vi "ge_DAQMain.vi"(8 "error in":errorcluster, 11 "DaqQ Name":string) -> (0 "error IO":errorcluster)   [LabVIEW 2012]
uses:
  Custom Ctrls/ge_TaskModBus.ctl
  Custom Ctrls/ge_AMC_Qname.ctl
  <resource>/objmgr/daqmx.rc
  Classes/Data Acquisition/Class DAQ Actor/DAQ Actor.lvclass
  Common/Controls/Group Timing Info.ctl
  Common/Controls/TE_Designator.ctl
  SubVIs Main/SubVIs DAQ/Custom Ctrls/ge_DAQBlockInfo.ctl
  SubVIs Main/SubVIs DAQ/Custom Ctrls/ge_DAQGrandmaster.ctl
  SubVIs Main/EZ Msg/ezm_Message.ctl
  <vilib>/DAQmx/read.llb/DAQmx Read (Analog 1D Wfm NChan NSamp).vi
  SubVIs Main/SubVIs DAQ/Custom Ctrls/ge_ThreadDiag.ctl
  <vilib>/addons/internet/NI_InternetTK_Core_VIs.lvlib
  Classes/Measurements/Class Channel/Channel.lvclass
panel:
  out "Numeric":i32
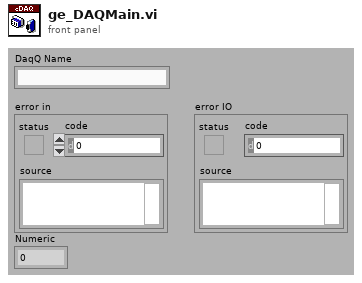
[diagram p1: front panel]
types:
  T1 = typedef "ge_DAQGrandmaster.ctl" = cluster{"Blocks ID":u32, "SisterThreadQName":string, "Chassis Name":string, "IP Address":string, "Speed":T2, "Backlog ID":string, "Backlog Enable":bool, "AllChans":refnum<class "Channel.lvclass">[], "ScalPrevNot":refnum<notifier>, "WfmPrevNot":refnum<notifier>, "DAQmx Task":refnum<k21>, "DS Conn":refnum<k13>, "DAQBlockInfo":T3, "TCP Wfm Queue":refnum<queue>, "UI Queue":refnum<queue>, "LS TCP Wfm Queue":refnum<queue>}
  T2 = typedef "TE_Designator.ctl" = enum16{"High Speed", "Low Speed"}
  T3 = typedef "ge_DAQBlockInfo.ctl" = cluster{"SampRate":dbl, "BufSize":u32, "ReadBlk":i32, "TCP Gap":i32}
  T4 = typedef "ge_AMC_Qname.ctl" = enum16{"Cmnd Loop", "UI Updater", "Conn Mgr HS", "Conn Mgr LS", "TCP Send HS", "TCP Send LS"}
  T5 = enum16{"Read", "Write", "ReadWrite", "BufferedRead", "BufferedReadWrite"}
  T6 = typedef "ge_ThreadDiag.ctl" = cluster{"Loop It":i32, "LoopRate (ms)":u32, "Bff Bcklg":dbl}
  T7 = typedef "ge_TaskModBus.ctl" = cluster{"Modbus URL":string, "Task":refnum<k21>, "IP Address":string, "GrpCfg":T8}
  T8 = typedef "Group Timing Info.ctl" = cluster{"Rate":dbl, "ReadBlk":i32, "TCP Gap":i32}
  T9 = typedef "DAQ Task Role.ctl" = enum16{"Master", "Slave", "Stand Alone", "None"}
  T10 = typedef "Telnet Session.ctl" = refnum<k1>
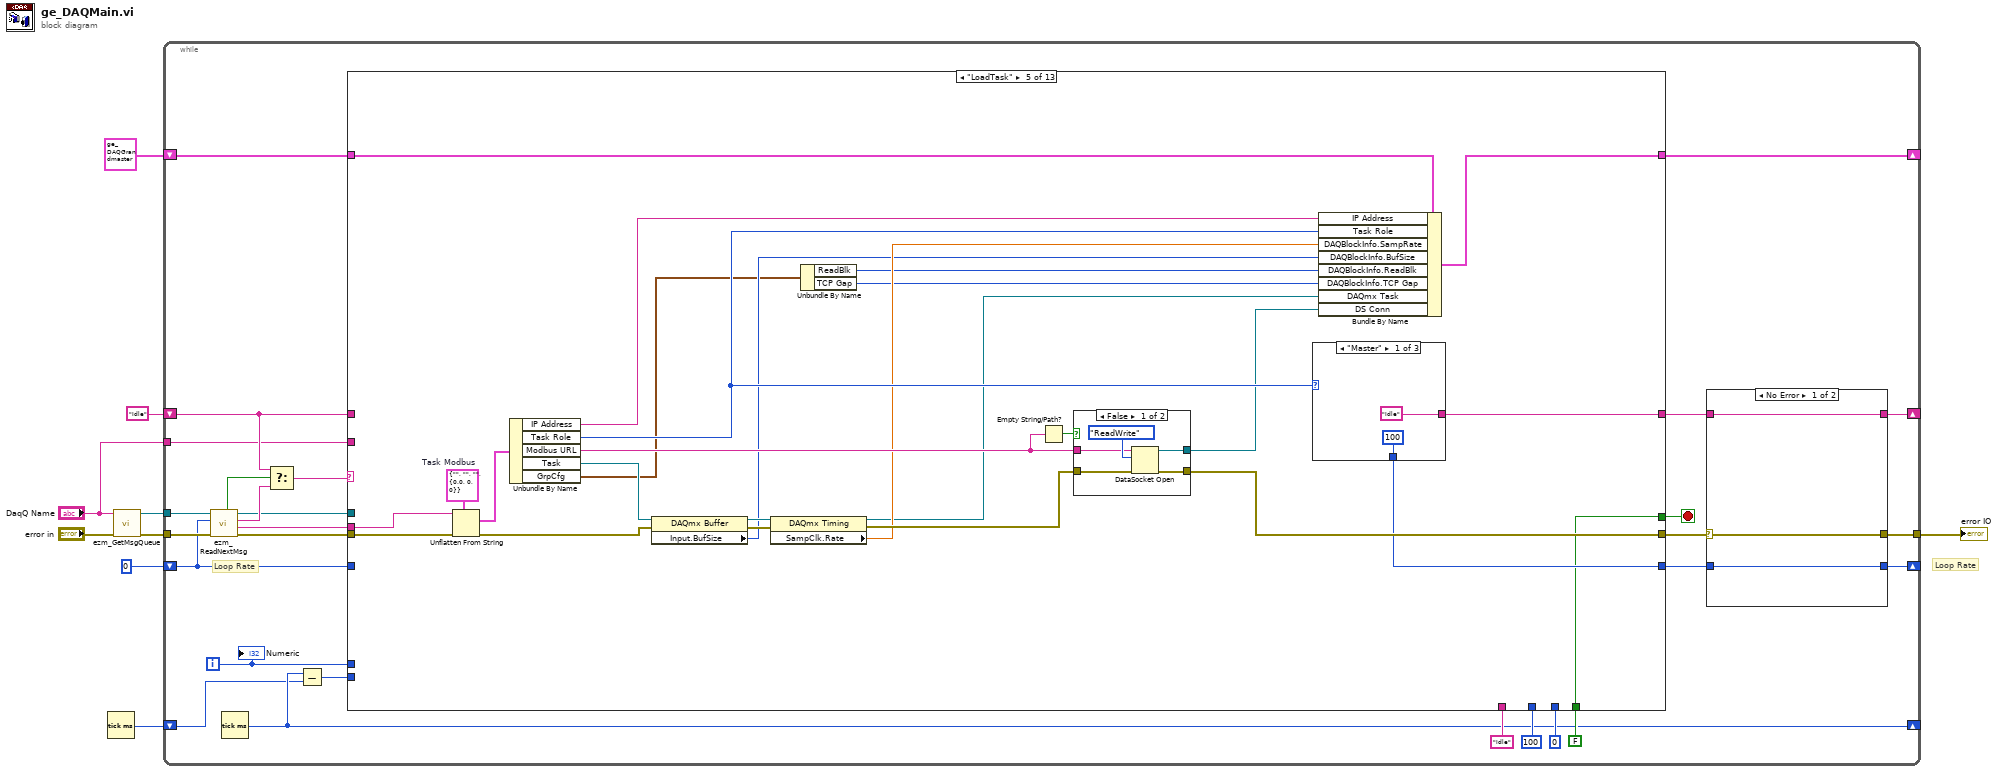
[diagram p0: block diagram]
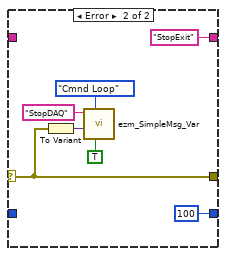
[diagram p2: hidden frame]
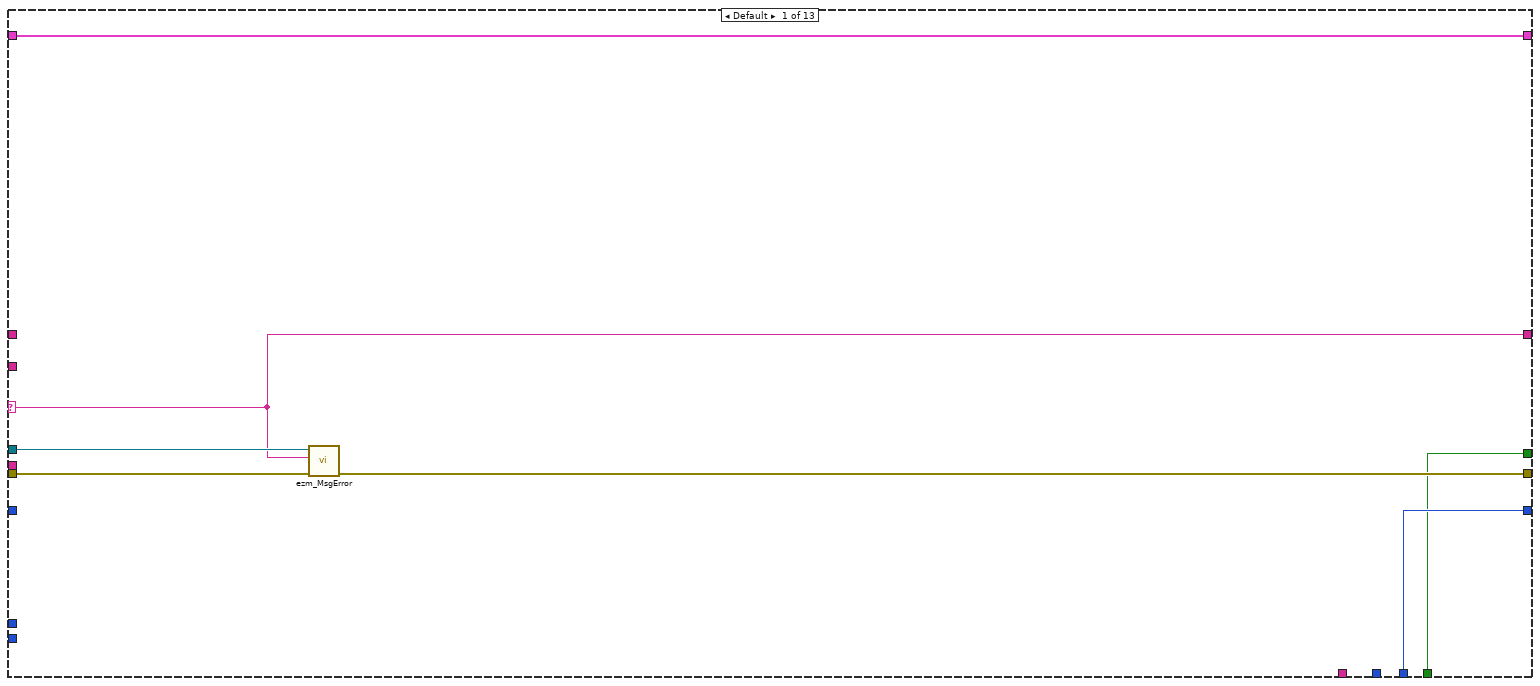
[diagram p3: hidden frame]
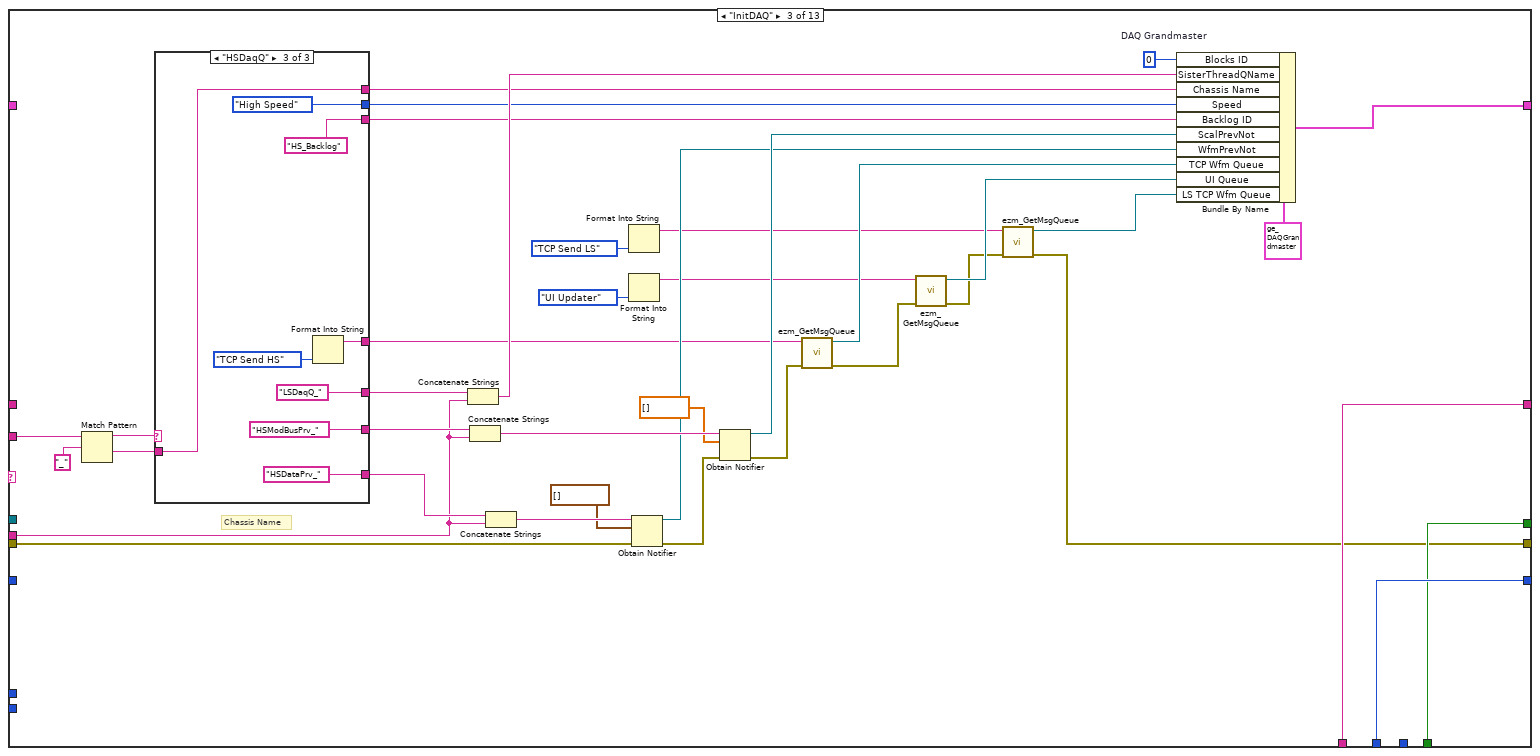
[diagram p5: hidden frame]
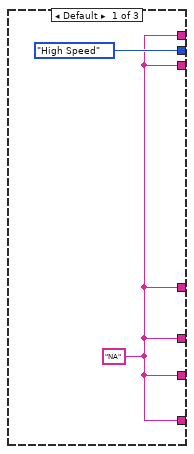
[diagram p6: hidden frame]
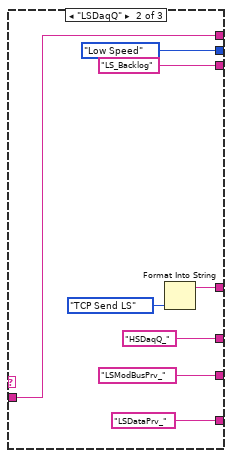
[diagram p7: hidden frame]
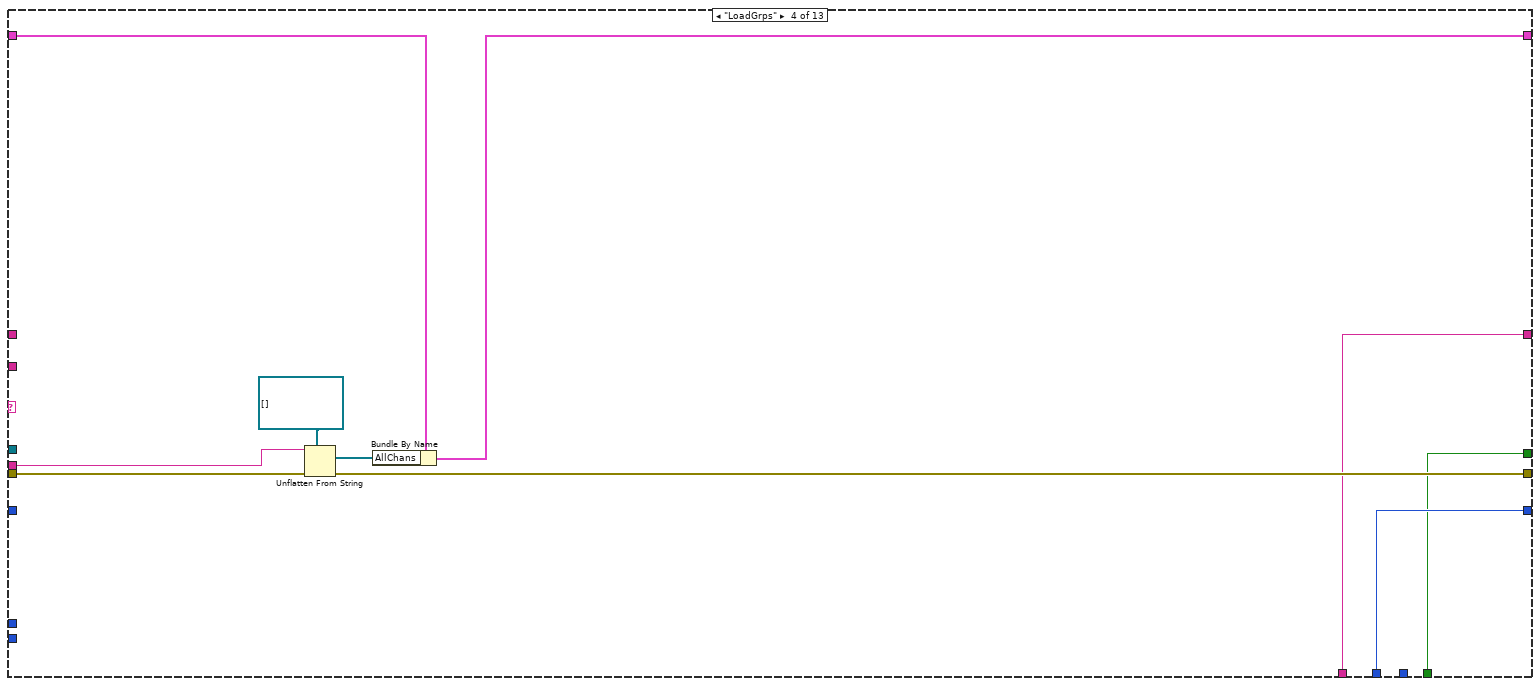
[diagram p8: hidden frame]
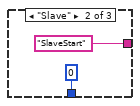
[diagram p9: hidden frame]
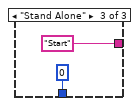
[diagram p10: hidden frame]
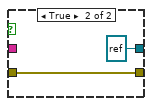
[diagram p11: hidden frame]
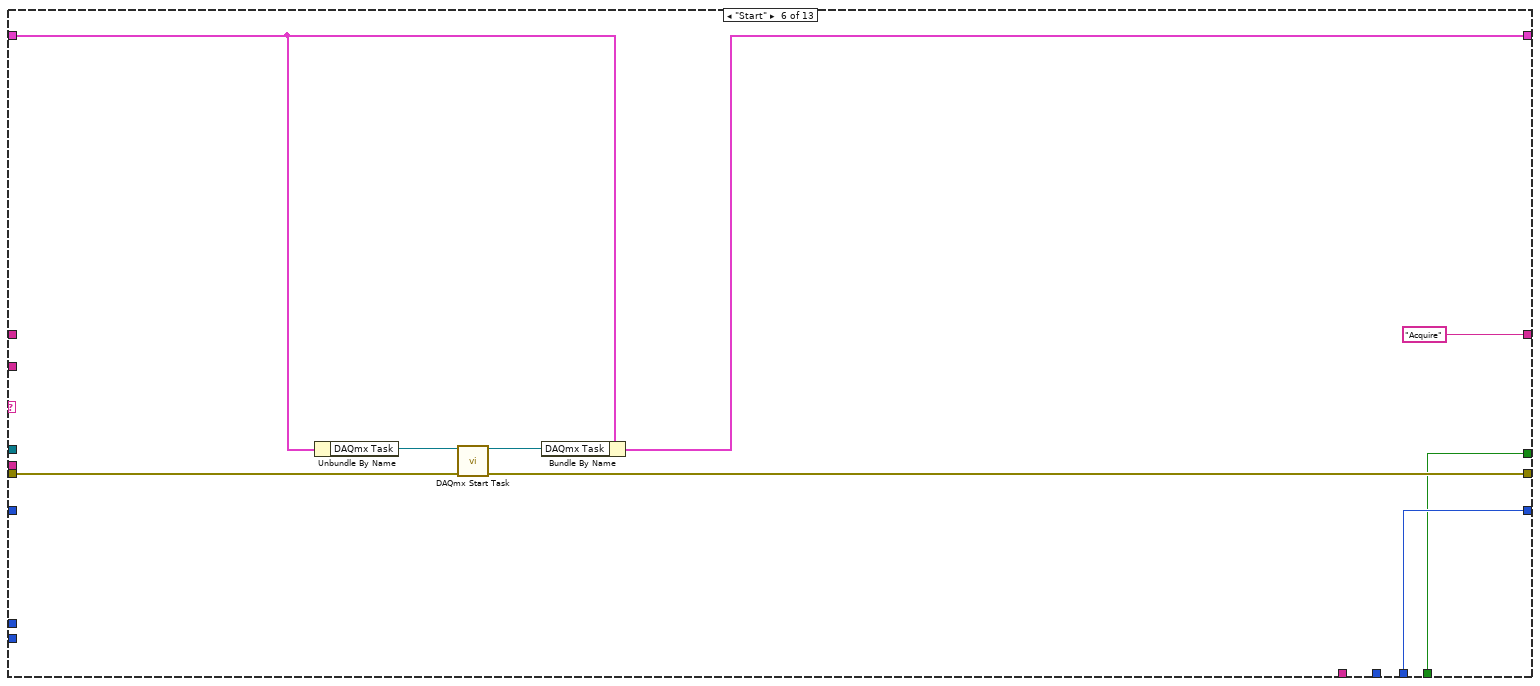
[diagram p12: hidden frame]
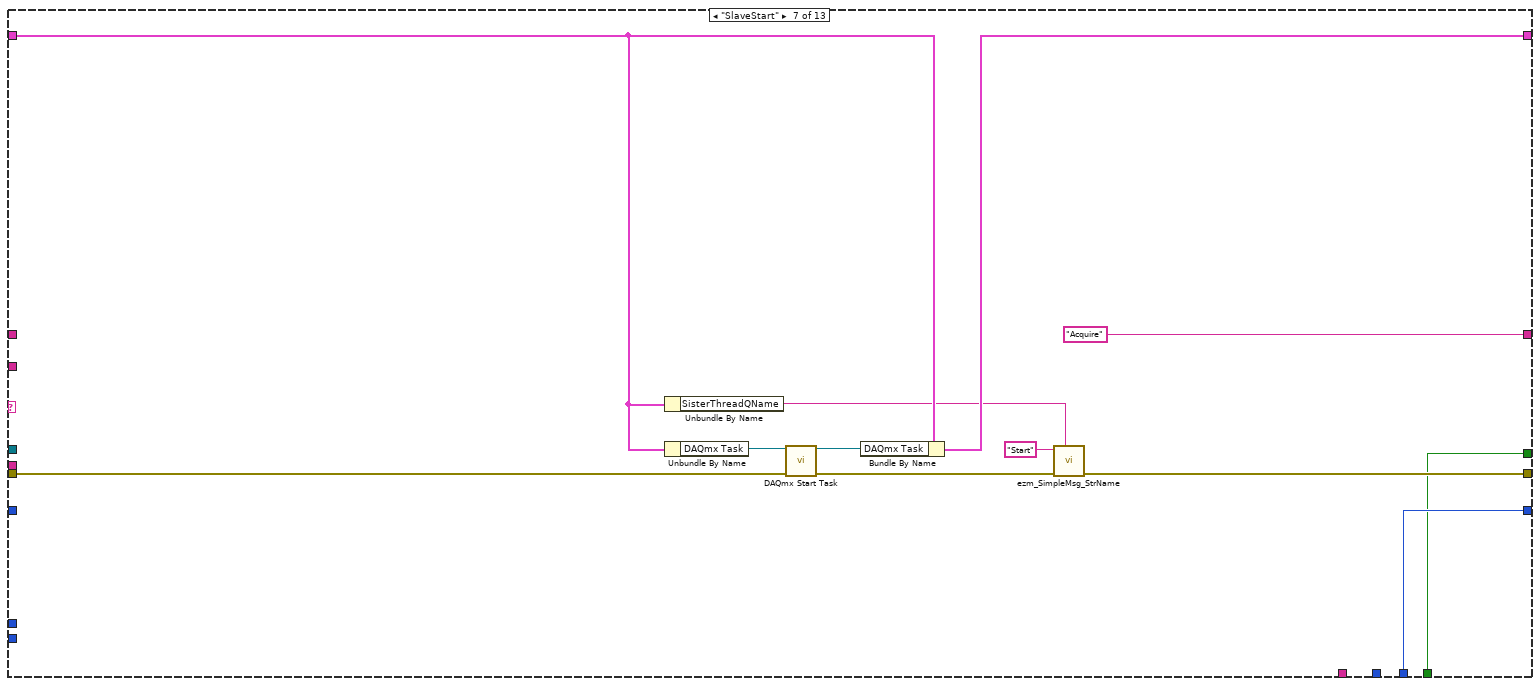
[diagram p13: hidden frame]
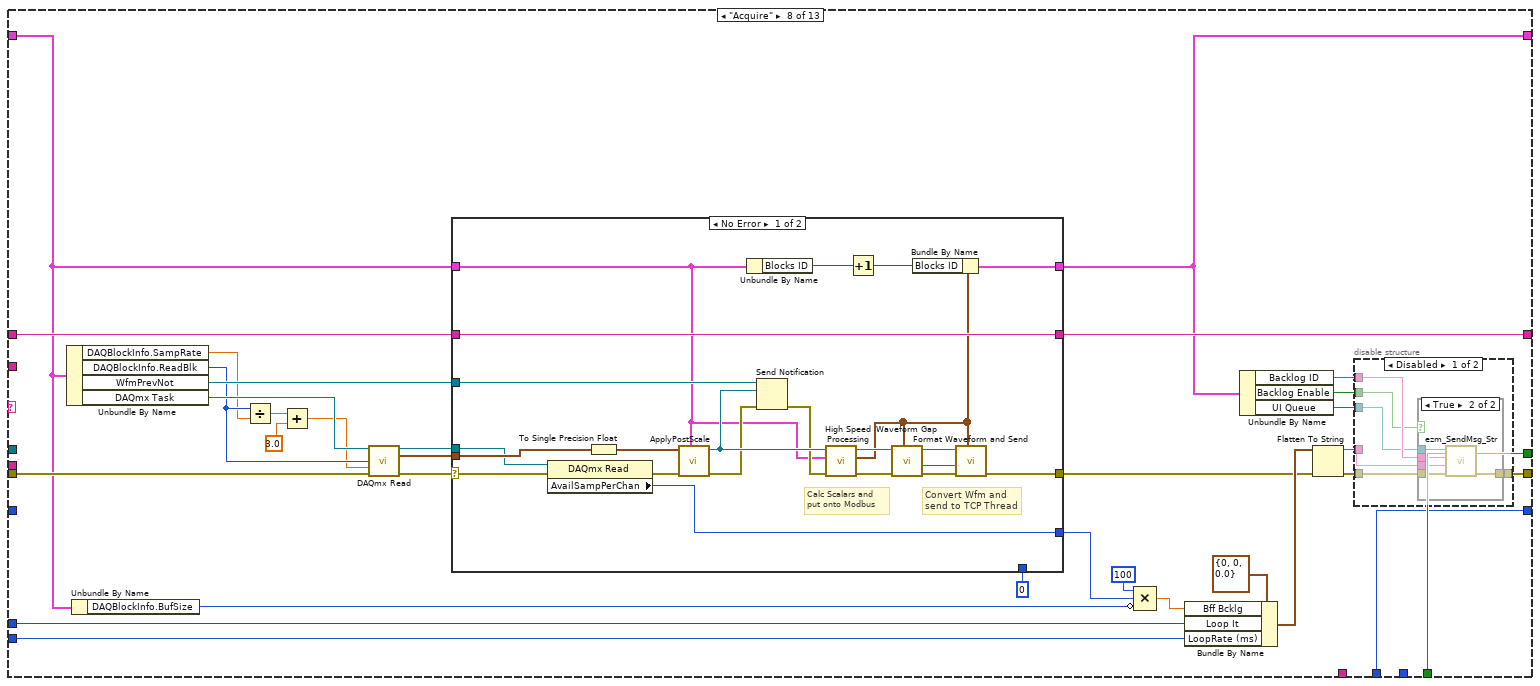
[diagram p14: hidden frame]
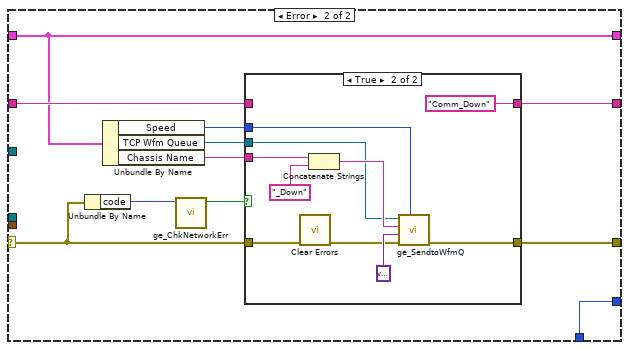
[diagram p17: hidden frame]
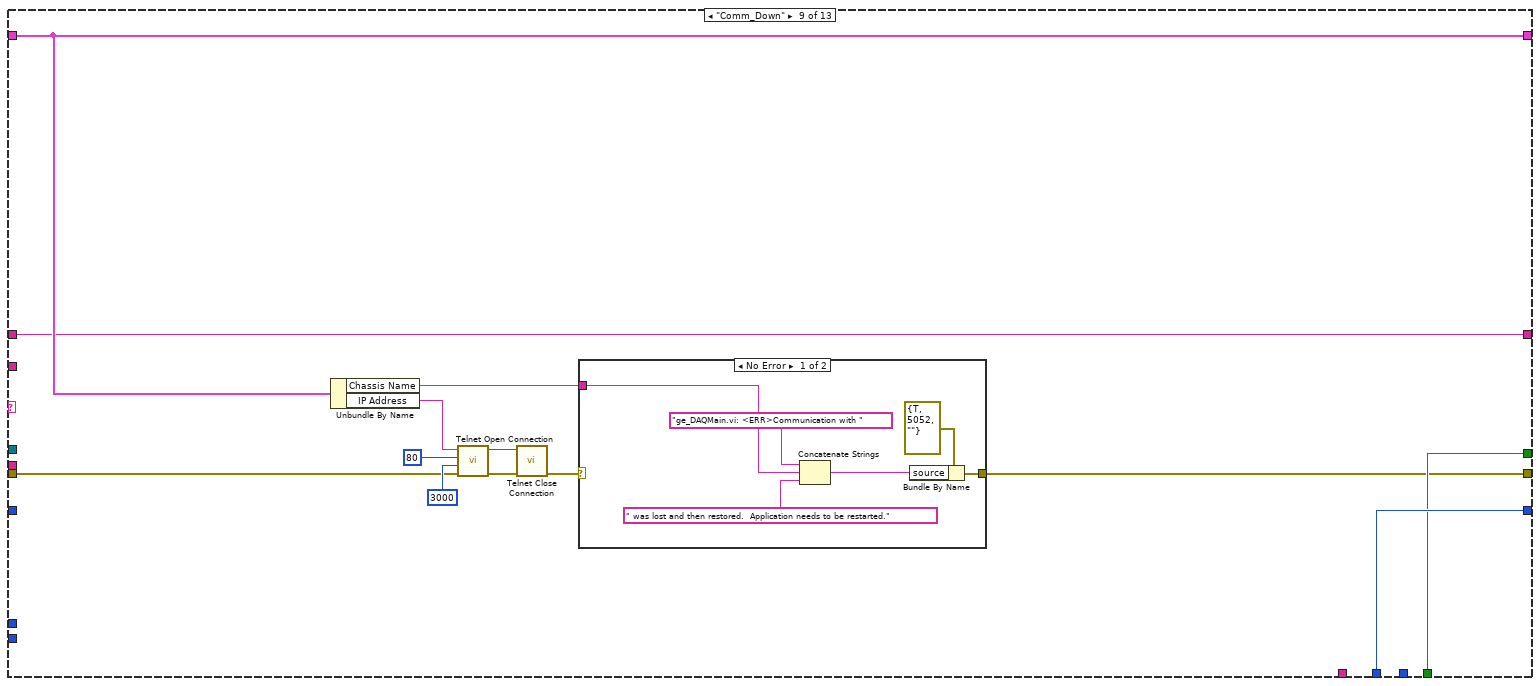
[diagram p19: hidden frame]
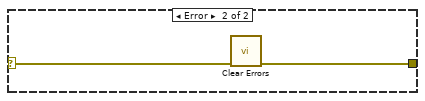
[diagram p20: hidden frame]
diagram:
  # "Loop Rate"
  n1 = Tick Count (ms)() -> (millisecond timer value=w3:u32)
  n2 = call "ezm_GetMsgQueue.vi"("error in"="error in", "Queue Name"="DaqQ Name") -> ("error out"=w6:errorcluster, "queue out"=w5:refnum<queue>)  [unwired: 8 in]
  n3 = while {
    tunnel: w6 -> [w36]
    tunnel: w5 -> [w37]
    shift-right: [w25] -> _
    shift-left: "Idle" ("Message Queue Name") -> [w21]
    shift-right: [w26] -> _
    shift-left: u32 0 -> [w30]
    tunnel: [w23] -> w2
    tunnel: "DaqQ Name" -> [w20]
    shift-right: [w15] -> _
    shift-left: T1 {"Blocks ID"=0, "SisterThreadQName"="", "Chassis Name"="", "IP Address"="", "Speed"=enum."High Speed", "Backlog ID"="", "Backlog Enable"=FALSE, "AllChans"=[], "ScalPrevNot"=refnum, "WfmPrevNot"=refnum, "DAQmx Task"="", "DS Conn"=refnum, "DAQBlockInfo"={"SampRate"=0.0, "BufSize"=0, "ReadBlk"=0, "TCP Gap"=0}, "TCP Wfm Queue"=refnum, "UI Queue"=refnum, "LS TCP Wfm Queue"=refnum} ("DAQ Grandmaster Out") -> [w14]
    shift-right: [w13] -> _
    shift-left: w3 -> [w12]
    i -> [w10]
    stop <- w17 stop-if-true
    # "Loop Rate"
    n4 = call "ezm_ReadNextMsg.vi"("error in"=w36, "timeout (0ms)"=w30, "Msg Queue In"=w37) -> ("error out"=w32:errorcluster, "Msg Value"=w33:string, "Msg Name"=w31:string, "Msg Queue Out"=w29:refnum<queue>, "timed out?"=w18:bool)  [unwired: 2 in, 2 out]
    n5 = Tick Count (ms)() -> (millisecond timer value=w13:u32)
    n6 = Select(t=w21, s=w18, f=w31) -> (s? t:f=w19:string)
    n7 = Subtract(x=w13, y=w12) -> (x-y=w11:u32)
    n8 = case shown="\"LoadTask\"" w19 {
      selector: w19 -> [w50 _ _ _ _ _ _ _ _ _ _ _ _]
      tunnel: w32 -> [w54 w59 w94 w124 w150 w173 w185 w209 w282 w303 w310 w329 w363]
      tunnel: [w53 w59 w63 w123 w141 w172 w182 w218 w287 w303 w310 w328 w383] -> w28
      tunnel: [w52 w58 w97 w121 w138 w170 w183 w203 w289 w302 w309 w324 u32 1000] -> w27
      tunnel: u32 0 -> [w52 _ _ _ _ w170 w183 _ _ _ _ w323 _]
      tunnel: w33 -> [_ _ w82 w125 w151 _ _ _ _ _ _ _ _]
      tunnel: u32 100 -> [_ w58 w97 w121 _ _ _ w203 w289 _ _ _ _]
      tunnel: [w50 w57 w90 w122 w148 "Acquire" ("Msg Name") "Acquire" ("Msg Name") w199 w285 w304 w311 w325 w382] -> w24
      tunnel: w30 -> [_ _ _ _ _ _ _ _ _ w302 w309 _ _]
      tunnel: w29 -> [w51 _ _ _ _ _ _ _ _ _ _ w330 w384]
      tunnel: "Idle" ("Msg Name") -> [_ w57 w90 w122 _ _ _ _ _ _ _ w326 w382]
      tunnel: w21 -> [_ _ _ _ _ _ _ w198 w285 w304 w311 w327 _]
      tunnel: w20 -> [_ _ w86 _ _ _ _ _ _ _ _ _ _]
      tunnel: [w49 w56 w81 w120 w137 w169 w179 w217 w288 w301 w308 w321 TRUE] -> w17
      tunnel: FALSE -> [w49 w56 w81 w120 w137 w169 w179 w217 w288 w301 w308 w322 _]
      tunnel: [w48 w55 w78 w118 w135 w165 w176 w190 w286 w298 w305 w320 w376] -> w15
      tunnel: w14 -> [w48 w55 _ w119 w136 w167 w175 w191 w286 w299 w306 w320 w376]
      tunnel: w11 -> [_ _ _ _ _ _ _ w212 _ _ _ _ _]
      tunnel: w10 -> [_ _ _ _ _ _ _ w210 _ _ _ _ _]
      frame Default {
        n9 = call "ezm_MsgError.vi"("error in"=w54, "AMC Msg Name"=w50, "Msg Queue"=w51) -> ("error out"=w53:errorcluster)  [unwired: 8 in]
      }
      frame "Idle" {
      }
      frame "InitDAQ" {
        w80 = T1 {"Blocks ID"=0, "SisterThreadQName"="", "Chassis Name"="", "IP Address"="", "Speed"=enum."High Speed", "Backlog ID"="", "Backlog Enable"=FALSE, "AllChans"=[], "ScalPrevNot"=refnum, "WfmPrevNot"=refnum, "DAQmx Task"="", "DS Conn"=refnum, "DAQBlockInfo"={"SampRate"=0.0, "BufSize"=0, "ReadBlk"=0, "TCP Gap"=0}, "TCP Wfm Queue"=refnum, "UI Queue"=refnum, "LS TCP Wfm Queue"=refnum}  # DAQ Grandmaster
        # "Chassis Name"
        n10 = Match Pattern(string=w86, regular expression="_") -> (before substring=w85:string, after substring=w84:string)  [unwired: 1 in, 2 out]
        n11 = case shown="\"HSDaqQ\"" w85 {
          tunnel: [w98 "LS_Backlog" ("Msg Name") "HS_Backlog" ("Msg Name")] -> w72
          tunnel: [w98 "LSModBusPrv_" ("name (unnamed)") "HSModBusPrv_" ("name (unnamed)")] -> w89
          tunnel: [w98 "LSDataPrv_" ("name (unnamed)") "HSDataPrv_" ("name (unnamed)")] -> w88
          tunnel: w84 -> [_ w103 w111]
          tunnel: [w98 w103 w111] -> w73
          tunnel: [TE_Designator."High Speed" ("Rate") TE_Designator."Low Speed" ("Rate") TE_Designator."High Speed" ("Rate")] -> w76
          tunnel: [w98 "HSDaqQ_" "LSDaqQ_"] -> w83
          tunnel: [w98 w100 w108] -> w69
          frame Default {
            w98 = "NA" ("Msg Name")
          }
          frame "LSDaqQ" {
            n12 = Format Into String(ge_AMC_Qname."TCP Send LS" ("ge_AMC_Qname")) -> (resulting string=w100:string)  [unwired: 3 in, 1 out]
          }
          frame "HSDaqQ" {
            n13 = Format Into String(ge_AMC_Qname."TCP Send HS" ("ge_AMC_Qname")) -> (resulting string=w108:string)  [unwired: 3 in, 1 out]
          }
        }
        n14 = Concatenate Strings(w83, w82) -> (w77:string)
        n15 = Concatenate Strings(w89, w82) -> (w92:string)
        n16 = Concatenate Strings(w88, w82) -> (w96:string)
        n17 = Format Into String(ge_AMC_Qname."TCP Send LS" ("ge_AMC_Qname")) -> (resulting string=w61:string)  [unwired: 3 in, 1 out]
        n18 = Format Into String(ge_AMC_Qname."UI Updater" ("ge_AMC_Qname")) -> (resulting string=w67:string)  [unwired: 3 in, 1 out]
        n19 = Obtain Notifier(name (unnamed)=w96, notification data type=waveform(sgl)[] [] ("data"), error in (no error)=w94) -> (notifier out=w74:refnum<notifier>, error out=w93:errorcluster)  [unwired: 1 in, 1 out]
        n20 = Obtain Notifier(name (unnamed)=w92, notification data type=dbl[] [], error in (no error)=w93) -> (notifier out=w75:refnum<notifier>, error out=w71:errorcluster)  [unwired: 1 in, 1 out]
        n21 = call "ezm_GetMsgQueue.vi"("error in"=w71, "Queue Name"=w69) -> ("error out"=w66:errorcluster, "queue out"=w70:refnum<queue>)  [unwired: 8 in]
        n22 = call "ezm_GetMsgQueue.vi"("error in"=w66, "Queue Name"=w67) -> ("error out"=w64:errorcluster, "queue out"=w65:refnum<queue>)  [unwired: 8 in]
        n23 = call "ezm_GetMsgQueue.vi"("error in"=w64, "Queue Name"=w61) -> ("error out"=w63:errorcluster, "queue out"=w60:refnum<queue>)  [unwired: 8 in]
        n24 = Bundle By Name(cluster=w80, "Blocks ID"=u32 0, "SisterThreadQName"=w77, "Chassis Name"=w73, "Speed"=w76, "Backlog ID"=w72, "ScalPrevNot"=w75, "WfmPrevNot"=w74, "TCP Wfm Queue"=w70, "UI Queue"=w65, "LS TCP Wfm Queue"=w60) -> (w78:T1)
      }
      frame "LoadGrps" {
        n25 = Unflatten From String(type=refnum<class "Channel.lvclass">[] [] ("AllChans"), binary string=w125, error in (no error)=w124) -> (value=w116:refnum<class "Channel.lvclass">[], error out=w123:errorcluster)  [unwired: 2 in, 1 out]
        n26 = Bundle By Name(cluster=w119, "AllChans"=w116) -> (w118:T1)
      }
      frame "LoadTask" {
        w149 = T7 {"Modbus URL"="", "Task"="", "IP Address"="", "GrpCfg"={"Rate"=0.0, "ReadBlk"=0, "TCP Gap"=0}}  # Task Modbus
        n27 = Unflatten From String(type=w149, binary string=w151, error in (no error)=w150) -> (value=w144:T7, error out=w143:errorcluster)  [unwired: 2 in, 1 out]
        n28 = Unbundle By Name(w144) -> ("IP Address"=w126:string, "Task Role"=w134:T9, "Modbus URL"=w139:string, "Task"=w145:refnum<k21>, "GrpCfg"=w131:T8)
        n29 = property class="DAQmx Buffer"(reference=w145, error in=w143) -> (reference out=w147:refnum<k21>, error out=w146:errorcluster, "Input.BufSize"=w132:u32)
        n30 = property class="DAQmx Timing"(reference=w147, error in=w146) -> (reference out=w128:refnum<k21>, error out=w142:errorcluster, "SampClk.Rate"=w133:dbl)
        n31 = Unbundle By Name(w131) -> ("ReadBlk"=w130:i32, "TCP Gap"=w129:i32)
        n32 = Empty String/Path?(string/path=w139) -> (empty?=w140:bool)
        n33 = case shown="False" w140 {
          tunnel: w142 -> [w161 w164]
          tunnel: [w160 w164] -> w141
          tunnel: w139 -> [w159 _]
          tunnel: [w158 refnum<k13> refnum ("connection id")] -> w127
          frame False {
            n34 = DataSocket Open(8:w161, 10:T5."ReadWrite" ("mode"), 11:w159) -> (0:w160:errorcluster, 3:w158:refnum<k13>)  [unwired: 1 in]
          }
          frame True {
          }
        }
        n35 = case shown="\"Master\"" w134 {
          tunnel: ["Idle" "SlaveStart" "Start"] -> w148
          tunnel: [u32 100 u32 0 u32 0] -> w138
          frame "Master" {
          }
          frame "Slave" {
          }
          frame "Stand Alone" {
          }
        }
        n36 = Bundle By Name(cluster=w136, "IP Address"=w126, "Task Role"=w134, "DAQBlockInfo.SampRate"=w133, "DAQBlockInfo.BufSize"=w132, "DAQBlockInfo.ReadBlk"=w130, "DAQBlockInfo.TCP Gap"=w129, "DAQmx Task"=w128, "DS Conn"=w127) -> (w135:T1)
      }
      frame "Start" {
        n37 = Unbundle By Name(w167) -> ("DAQmx Task"=w168:refnum<k21>)
        n38 = call <vilib>:"DAQmx Start Task.vi"("task/channels in"=w168, "error in"=w173) -> ("task out"=w166:refnum<k21>, "error out"=w172:errorcluster)  [unwired: 12 in]
        n39 = Bundle By Name(cluster=w167, "DAQmx Task"=w166) -> (w165:T1)
      }
      frame "SlaveStart" {
        n40 = Unbundle By Name(w175) -> ("SisterThreadQName"=w174:string)
        n41 = Unbundle By Name(w175) -> ("DAQmx Task"=w178:refnum<k21>)
        n42 = call <vilib>:"DAQmx Start Task.vi"("task/channels in"=w178, "error in"=w185) -> ("task out"=w177:refnum<k21>, "error out"=w181:errorcluster)  [unwired: 12 in]
        n43 = Bundle By Name(cluster=w175, "DAQmx Task"=w177) -> (w176:T1)
        n44 = call "ezm_SimpleMsg_StrName.vi"("Destination Queue"=w174, "error in"=w181, "Msg Name"="Start" ("Message Name")) -> ("error out"=w182:errorcluster)  [unwired: 7 in, 1 out]
      }
      frame "Acquire" {
        n45 = Unbundle By Name(w191) -> ("DAQBlockInfo.SampRate"=w196:dbl, "DAQBlockInfo.ReadBlk"=w197:i32, "WfmPrevNot"=w204:refnum<notifier>, "DAQmx Task"=w205:refnum<k21>)
        n46 = Unbundle By Name(w191) -> ("DAQBlockInfo.BufSize"=w208:u32)
        n47 = Divide(x=w197, y=w196) -> (x/y=w195:dbl)
        n48 = Add(x=w195, y=3.0) -> (x+y=w193:dbl)
        n49 = call-poly <vilib>:"DAQmx Read.vi"("task/channels in"=w205, "number of samples per channel"=w197, "timeout"=w193, "error in"=w209) -> ("task out"=w201:refnum<k21>, "data"=w202:waveform(dbl)[], "error out"=w200:errorcluster)  [unwired: 9 in]
        n50 = case shown="No Error" w200 {
          selector: w200 -> [w238 w262]
          tunnel: [w253 w258] -> w186
          tunnel: [w252 w261] -> w206
          tunnel: w204 -> [w251 _]
          tunnel: w191 -> [w234 w254]
          tunnel: w202 -> [w250 _]
          tunnel: w201 -> [w248 _]
          tunnel: [w237 w264] -> w199
          tunnel: w198 -> [w237 w259]
          tunnel: u32 0 ("AvailSampPerChan") -> [_ w258]
          tunnel: [w232 w254] -> w190
          frame No Error {
            # "Convert Wfm and\nsend to TCP Thread"
            # "Calc Scalars and\nput onto Modbus"
            n51 = property class="DAQmx Read"(reference=w248, error in=w238) -> (error out=w246:errorcluster, "AvailSampPerChan"=w253:u32)  [unwired: 1 out]
            n52 = To Single Precision Float(number=w250) -> (single precision float=w247:waveform(sgl)[])
            n53 = call "ApplyPostScale.vi"(7:w234, "error in (no error)"=w246, "DAQ Actor in"=w247) -> ("error out"=w240:errorcluster, "DAQ Actor Out"=w241:refnum<class "DAQ Actor.lvclass">)  [unwired: 6 in, 1 out]
            n54 = Unbundle By Name(w234) -> ("Blocks ID"=w236:u32)
            n55 = Send Notification(notification=w241, notifier=w251, error in (no error)=w240) -> (error out=w239:errorcluster)  [unwired: 1 out]
            n56 = call "High Speed Processing.vi"("error in"=w239, "Wfm data"=w234, "DAQ Actor in"=w241) -> ("error out"=w245:errorcluster, "Wfm out"=w233:waveform(sgl)[], "DAQ Actor out"=w244:refnum<class "DAQ Actor.lvclass">)  [unwired: 6 in]
            n57 = Increment(x=w236) -> (x+1=w235:u32)
            n58 = call "Waveform Gap.vi"(7:w233, "error in"=w245, "DAQ Actor in"=w244) -> ("error out"=w249:errorcluster, "Output Block"=w243:bool, "DAQ Actor out"=w242:refnum<class "DAQ Actor.lvclass">)  [unwired: 5 in, 1 out]
            n59 = Bundle By Name(cluster=w233, "Blocks ID"=w235) -> (w232:cluster{})
            n60 = call "Format Waveform and Send.vi"(7:w233, "error in (no error)"=w249, "Output Block"=w243, "DAQ Actor in"=w242) -> ("error out"=w252:errorcluster)  [unwired: 6 in, 1 out]
          }
          frame Error {
            n61 = Unbundle By Name(w262) -> ("code"=w263:i32)
            n62 = Unbundle By Name(w254) -> ("Speed"=w257:T2, "TCP Wfm Queue"=w256:refnum<queue>, "Chassis Name"=w255:string)
            n63 = call "ge_ChkNetworkErr.vi"("Error Code"=w263) -> ("Network Error?"=w260:bool)  [unwired: 10 in]
            n64 = case shown="True" w260 {
              tunnel: [w265 "Comm_Down"] -> w264
              tunnel: w262 -> [w266 w275]
              tunnel: [w266 w270] -> w261
              tunnel: w259 -> [w265 _]
              tunnel: w257 -> [_ w269]
              tunnel: w255 -> [_ w268]
              tunnel: w256 -> [_ w267]
              frame False {
              }
              frame True {
                n65 = call <vilib>:"Clear Errors.vi"("error in (no error)"=w275) -> ("error out"=w271:errorcluster)  [unwired: 6 in]
                n66 = Concatenate Strings(w268, "_Down" ("string")) -> (w273:string)
                n67 = call "ge_SendtoWfmQ.vi"("Rate"=w269, "error in"=w271, "variant"=variant, "Metadata"=w273, "Msg Queue In"=w267) -> ("error out"=w270:errorcluster)  [unwired: 6 in]
              }
            }
          }
        }
        n68 = Compound Arithmetic op=MULTIPLY(u32 100 ("value"), w186, invert w208) -> (w189:dbl)
        n69 = Bundle By Name(cluster=T6 {"Loop It"=0, "LoopRate (ms)"=0, "Bff Bcklg"=0.0} ("ThreadDiag"), "Bff Bcklg"=w189, "Loop It"=w210, "LoopRate (ms)"=w212) -> (w211:T6)
        n70 = Unbundle By Name(w190) -> ("Backlog ID"=w216:string, "Backlog Enable"=w215:bool, "UI Queue"=w213:refnum<queue>)
        n71 = Flatten To String(anything=w211, error in (no error)=w206) -> (data string=w214:string, error out=w207:errorcluster)  [unwired: 2 in, 1 out]
        n72 = disable-structure shown="Disabled" {
          disable-tunnel: [w224 w231] -> w218
          disable-tunnel: w216 -> [w223 _]
          disable-tunnel: w215 -> [w222 _]
          disable-tunnel: w214 -> [w221 _]
          disable-tunnel: w213 -> [w220 _]
          disable-tunnel: w207 -> [w219 w231]
          frame Disabled {
            n73 = case shown="True" w222 {
              tunnel: [w225 w229] -> w224
              tunnel: w219 -> [w225 w230]
              tunnel: w223 -> [_ w228]
              tunnel: w221 -> [_ w227]
              tunnel: w220 -> [_ w226]
              frame False {
              }
              frame True {
                n74 = call "ezm_SendMsg_Str.vi"("error in"=w230, "Msg Value"=w227, "Msg Name"=w228, "Msg Queue In"=w226) -> ("error out"=w229:errorcluster)  [unwired: 4 in, 3 out]
              }
            }
          }
          frame Enabled {
          }
        }
      }
      frame "Comm_Down" {
        n75 = Unbundle By Name(w286) -> ("Chassis Name"=w279:string, "IP Address"=w277:string)
        n76 = call <vilib>:"Telnet Open Connection.vi"("error in (no error)"=w282, "timeout ms (60000)"=3000, "remote port (23)"=u16 80, "address"=w277) -> ("error out"=w283:errorcluster, "telnet connection"=w280:T10)  [unwired: 6 in]
        n77 = call <vilib>:"Telnet Close Connection.vi"("error in (no error)"=w283, "telnet connection"=w280) -> ("error out"=w281:errorcluster)  [unwired: 8 in, 1 out]
        n78 = case shown="No Error" w281 {
          selector: w281 -> [_ w297]
          tunnel: [w291 w296] -> w287
          tunnel: w279 -> [w290 _]
          frame No Error {
            n79 = Concatenate Strings("ge_DAQMain.vi: <ERR>Communication with ", w290, " was lost and then restored.  Application needs to be restarted.") -> (w292:string)
            n80 = Bundle By Name(cluster=errorcluster {"status"=TRUE, "code"=5052, "source"=""} ("error IO"), "source"=w292) -> (w291:errorcluster)
          }
          frame Error {
            n81 = call <vilib>:"Clear Errors.vi"("error in (no error)"=w297) -> ("error out"=w296:errorcluster)  [unwired: 6 in]
          }
        }
      }
      frame "EnableBacklog" {
        n82 = Bundle By Name(cluster=w299, "Backlog Enable"=TRUE) -> (w298:T1)
      }
      frame "DisableBacklog" {
        n83 = Bundle By Name(cluster=w306, "Backlog Enable"=FALSE) -> (w305:T1)
      }
      frame "StopExit" {
        n84 = Unbundle By Name(w320) -> ("Task Role"=w316:T9, "SisterThreadQName"=w319:string, "ScalPrevNot"=w318:refnum<notifier>, "WfmPrevNot"=w317:refnum<notifier>, "DS Conn"=w315:refnum<k13>, "TCP Wfm Queue"=w314:refnum<queue>, "UI Queue"=w313:refnum<queue>, "LS TCP Wfm Queue"=w312:refnum<queue>)
        n85 = case shown="\"Slave\", \"Stand Alone\"" w316 {
          tunnel: w330 -> [_ w355]
          tunnel: w329 -> [w334 w335]
          tunnel: w318 -> [_ w354]
          tunnel: w317 -> [_ w353]
          tunnel: [w334 w352] -> w328
          tunnel: w319 -> [_ w351]
          tunnel: w316 -> [_ w350]
          tunnel: w315 -> [_ w346]
          tunnel: w327 -> [w333 _]
          tunnel: w326 -> [_ w345]
          tunnel: [w333 w345] -> w325
          tunnel: [w332 u32 1000] -> w324
          tunnel: w323 -> [w332 _]
          tunnel: [w331 TRUE] -> w321
          tunnel: w322 -> [w331 _]
          tunnel: w314 -> [_ w341]
          tunnel: w313 -> [_ w339]
          tunnel: w312 -> [_ w336]
          frame "Master" {
          }
          frame "Slave", "Stand Alone" {
            n86 = case shown="\"Slave\"" w350 {
              tunnel: w335 -> [w356 w359]
              tunnel: [w356 w360] -> w347
              tunnel: w351 -> [_ w357]
              frame Default {
              }
              frame "Slave" {
                n87 = call "ezm_SimpleMsg_StrName.vi"("Destination Queue"=w357, "error in"=w359, "Msg Name"="MasterStopExit" ("Message Name")) -> ("error out"=w360:errorcluster)  [unwired: 7 in, 1 out]
              }
            }
            n88 = Release Notifier(notifier=w354, error in (no error)=w347) -> (error out=w349:errorcluster)  [unwired: 1 in, 2 out]
            n89 = Release Notifier(notifier=w353, error in (no error)=w349) -> (error out=w348:errorcluster)  [unwired: 1 in, 2 out]
            n90 = DataSocket Close(8:w348, 11:w346) -> (0:w342:errorcluster)  [unwired: 1 in, 1 out]
            n91 = Release Queue(queue=w341, error in (no error)=w342) -> (error out=w340:errorcluster)  [unwired: 1 in, 2 out]
            n92 = Release Queue(queue=w339, error in (no error)=w340) -> (error out=w338:errorcluster)  [unwired: 1 in, 2 out]
            n93 = Release Queue(queue=w336, error in (no error)=w338) -> (error out=w337:errorcluster)  [unwired: 1 in, 2 out]
            n94 = flat-sequence {
              tunnel: w355 -> [w361]
              tunnel: [errorcluster {"status"=FALSE, "code"=0, "source"=""} ("error out")] -> w352
              tunnel: w337 -> [_]
              frame #0 {
                n95 = call "ezm_DestroyQueue.vi"("Queue in"=w361) -> ()  [unwired: 10 in, 1 out]
              }
            }
          }
        }
      }
      frame "MasterStopExit" {
        # "When in a synchronized case, we must stop the slave first and then the master.\nIf you just send \"Exit\" to all threads regardless of role, the slave threads SOMETIMES timeout.\nTo prevent this filter the stop commands to make sure the slaves stop and then have the slaves send stop to the masters."
        n96 = Unbundle By Name(w376) -> ("Task Role"=w375:T9, "SisterThreadQName"=w374:string, "ScalPrevNot"=w373:refnum<notifier>, "WfmPrevNot"=w372:refnum<notifier>, "DS Conn"=w371:refnum<k13>, "TCP Wfm Queue"=w369:refnum<queue>, "UI Queue"=w367:refnum<queue>, "LS TCP Wfm Queue"=w364:refnum<queue>)
        n97 = case shown="\"Slave\"" w375 {
          tunnel: w363 -> [w385 w388]
          tunnel: [w385 w389] -> w378
          tunnel: w374 -> [_ w386]
          frame Default {
          }
          frame "Slave" {
            n98 = call "ezm_SimpleMsg_StrName.vi"("Destination Queue"=w386, "error in"=w388, "Msg Name"="MasterStopExit" ("Message Name")) -> ("error out"=w389:errorcluster)  [unwired: 7 in, 1 out]
          }
        }
        n99 = Release Notifier(notifier=w373, error in (no error)=w378) -> (error out=w380:errorcluster)  [unwired: 1 in, 2 out]
        n100 = Release Notifier(notifier=w372, error in (no error)=w380) -> (error out=w379:errorcluster)  [unwired: 1 in, 2 out]
        n101 = DataSocket Close(8:w379, 11:w371) -> (0:w370:errorcluster)  [unwired: 1 in, 1 out]
        n102 = Release Queue(queue=w369, error in (no error)=w370) -> (error out=w368:errorcluster)  [unwired: 1 in, 2 out]
        n103 = Release Queue(queue=w367, error in (no error)=w368) -> (error out=w366:errorcluster)  [unwired: 1 in, 2 out]
        n104 = Release Queue(queue=w364, error in (no error)=w366) -> (error out=w365:errorcluster)  [unwired: 1 in, 2 out]
        n105 = flat-sequence {
          tunnel: w384 -> [w390]
          tunnel: [errorcluster {"status"=FALSE, "code"=0, "source"=""} ("error out")] -> w383
          tunnel: w365 -> [_]
          frame #0 {
            n106 = call "ezm_DestroyQueue.vi"("Queue in"=w390) -> ()  [unwired: 10 in, 1 out]
          }
        }
      }
    }
    n107 = case shown="No Error" w28 {
      selector: w28 -> [w38 w41]
      tunnel: [w40 "StopExit" ("Msg Name")] -> w25
      tunnel: w24 -> [w40 _]
      tunnel: w27 -> [w39 _]
      tunnel: [w39 u32 100] -> w26
      tunnel: [w38 w41] -> w23
      frame No Error {
      }
      frame Error {
        n108 = To Variant(anything=w41) -> (Variant=w42:variant)
        n109 = call "ezm_SimpleMsg_Var.vi"("Priority Message (F)"=TRUE, "Destination Queue"=ge_AMC_Qname."Cmnd Loop" ("ge_AMC_Qname"), "Msg Data"=w42, "Msg Name"="StopDAQ") -> ()  [unwired: 6 in, 2 out]
      }
    }
    "Numeric" <- w10
  }
  "error IO" <- w2
